vi "SetCurrent.vi"(3 "Current":dbl step=1.0 format="%.3f", 4 "error in":errorcluster, 5 "connection ID":refnum<k5>) -> (0 "False":bool, 1 "error out":errorcluster, 2 "connection ID out":refnum<k5>)   [LabVIEW 2013]
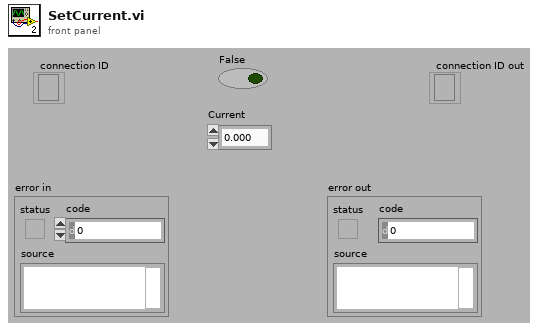
[diagram p1: front panel]
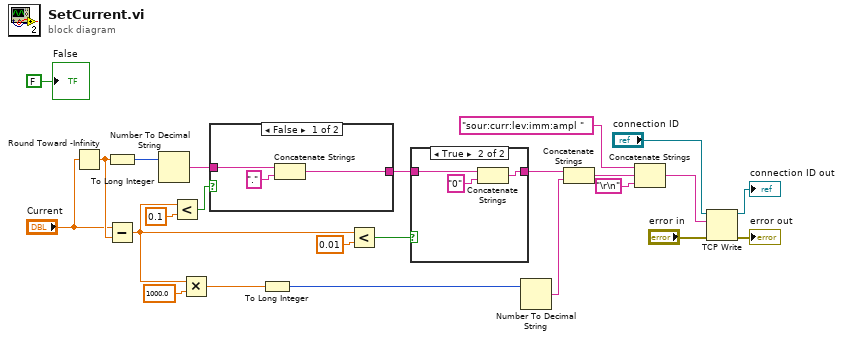
[diagram p0: block diagram]
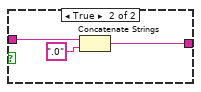
[diagram p3: hidden frame]
diagram:
  n1 = Round Toward -Infinity(1:"Current") -> (0:w16:dbl)
  n2 = To Long Integer(number=w16) -> (32bit integer=w14:i32)
  n3 = Subtract(x="Current", y=w16) -> (x-y=w10:dbl)
  n4 = Number To Decimal String(number=w14) -> (decimal integer string=w8:string)  [unwired: 1 out]
  n5 = Less?(x=w10, y=0.1) -> (x < y?=w9:bool)
  n6 = Multiply(x=w10, y=1000.0) -> (x*y=w17:dbl)
  n7 = case shown="False" w9 {
    tunnel: w8 -> [w26 w29]
    tunnel: [w25 w28] -> w6
    frame False {
      n8 = Concatenate Strings(w26, "." ("string")) -> (w25:string)
    }
    frame True {
      n9 = Concatenate Strings(w29, ".0" ("string")) -> (w28:string)
    }
  }
  n10 = To Long Integer(number=w17) -> (32bit integer=w15:i32)
  n11 = Less?(x=w10, y=0.01) -> (x < y?=w7:bool)
  n12 = case shown="True" w7 {
    tunnel: w6 -> [w31 w33]
    tunnel: [w31 w32] -> w5
    frame False {
    }
    frame True {
      n13 = Concatenate Strings(w33, "0" ("string")) -> (w32:string)
    }
  }
  n14 = Number To Decimal String(number=w15) -> (decimal integer string=w13:string)  [unwired: 1 out]
  n15 = Concatenate Strings(w5, w13) -> (w3:string)
  n16 = Concatenate Strings("sour:curr:lev:imm:ampl " ("data in"), w3, "\r\n") -> (w22:string)
  n17 = TCP Write(connection ID="connection ID", data in=w22, error in (no error)="error in") -> (connection ID out=→"connection ID out":refnum<k5>, error out=→"error out":errorcluster)  [unwired: 2 out]
  "False" <- FALSE
